vi "Simulation-06.vi"() -> (0 "error out":errorcluster, 3 "success":bool)   [LabVIEW 2020]
uses:
  librarian_class/typedefs/book_state--enum.ctl
  shared/request--enum.ctl
  librarian_class/librarian.lvclass
  client_class/client.lvclass
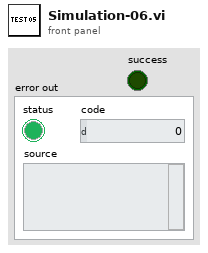
[diagram p1: front panel]
types:
  T1 = typedef "request--enum.ctl" = enum16{"CHECKIN", "CHECKOUT"}
  T2 = typedef "librarian.lvclass/book_state--enum.ctl" = enum16{"CHECKEDIN", "CHECKEDOUT", "DAMAGED"}
  T3 = typedef "message--cluster.ctl" = cluster{"header":string, "cmd":T1, "title":string, "book":string}
  T4 = typedef "librarian.lvclass/lib_map_value--cluster.ctl" = cluster{"book state":T2, "text":string, "hash":string}
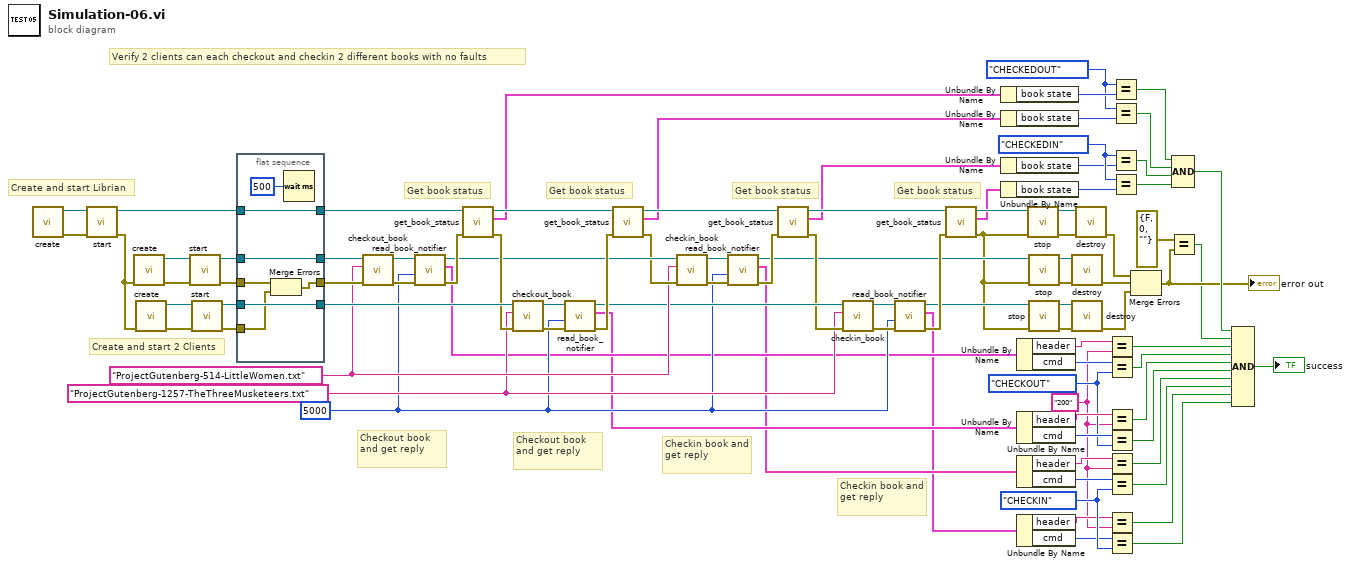
[diagram p0: block diagram]
diagram:
  w23 = request--enum."CHECKIN" ("y")
  w24 = request--enum."CHECKOUT" ("y")
  w18 = "200" ("x")
  w37 = book_state--enum."CHECKEDIN" ("x")
  w38 = book_state--enum."CHECKEDOUT" ("x")
  w58 = 5000 ("timeout in ms (-1)")
  w61 = "ProjectGutenberg-1257-TheThreeMusketeers.txt" ("book title")
  w68 = "ProjectGutenberg-514-LittleWomen.txt" ("book title")
  # "Verify 2 clients can each checkout and checkin 2 different books with no faults"
  # "Get book status"
  # "Get book status"
  # "Get book status"
  # "Get book status"
  # "Checkin book and get reply"
  # "Checkin book and get reply"
  # "Checkout book and get reply"
  # "Checkout book and get reply"
  # "Create and start 2 Clients"
  # "Create and start Librian"
  n1 = call "create.vi"() -> ("error out"=w93:errorcluster, "librarian_sm out"=w94:refnum<class "librarian.lvclass">)  [unwired: 10 in]
  n2 = call "start.vi"("error in (no error)"=w93, "librarian_sm in"=w94) -> ("error out"=w89:errorcluster, "librarian_sm out"=w88:refnum<class "librarian.lvclass">)  [unwired: 8 in]
  n3 = call "create.vi"("error in (no error)"=w89) -> ("error out"=w91:errorcluster, "librarian_sm out"=w92:refnum<class "client.lvclass">)  [unwired: 9 in]
  n4 = call "create.vi"("error in (no error)"=w89) -> ("error out"=w85:errorcluster, "librarian_sm out"=w90:refnum<class "client.lvclass">)  [unwired: 9 in]
  n5 = call "start.vi"("error in (no error)"=w91, "librarian_sm in"=w92) -> ("error out"=w87:errorcluster, "librarian_sm out"=w84:refnum<class "client.lvclass">)  [unwired: 8 in]
  n6 = call "start.vi"("error in (no error)"=w85, "librarian_sm in"=w90) -> ("error out"=w86:errorcluster, "librarian_sm out"=w83:refnum<class "client.lvclass">)  [unwired: 8 in]
  n7 = flat-sequence {
    tunnel: w88 -> [w101]
    tunnel: w87 -> [w97]
    tunnel: w86 -> [w96]
    tunnel: w84 -> [w100]
    tunnel: w83 -> [w99]
    tunnel: [w101] -> w75
    tunnel: [w100] -> w81
    tunnel: [w95] -> w80
    tunnel: [w99] -> w76
    frame #0 {
      n8 = Merge Errors(w97, w96) -> (w95:errorcluster)
      n9 = Wait (ms)(milliseconds to wait=u32 500) -> ()  [unwired: 1 out]
    }
  }
  n10 = call "checkout_book.vi"("error in (no error)"=w80, "book title"=w68, "client in"=w81) -> ("error out"=w79:errorcluster, "client out"=w82:refnum<class "client.lvclass">)  [unwired: 7 in]
  n11 = call "read_book_notifier.vi"("error in (no error)"=w79, "timeout in ms (-1)"=w58, "client in"=w82) -> ("error out"=w74:errorcluster, "msg"=w17:T3, "client out"=w70:refnum<class "client.lvclass">)  [unwired: 6 in]
  n12 = call "get_book_status.vi"("error in (no error)"=w74, "librarian in"=w75) -> ("error out"=w73:errorcluster, "book status"=w40:T4, "librarian out"=w72:refnum<class "librarian.lvclass">)  [unwired: 7 in]
  n13 = call "checkout_book.vi"("error in (no error)"=w73, "book title"=w61, "client in"=w76) -> ("error out"=w78:errorcluster, "client out"=w77:refnum<class "client.lvclass">)  [unwired: 7 in]
  n14 = call "read_book_notifier.vi"("error in (no error)"=w78, "timeout in ms (-1)"=w58, "client in"=w77) -> ("error out"=w71:errorcluster, "msg"=w16:T3, "client out"=w63:refnum<class "client.lvclass">)  [unwired: 6 in]
  n15 = call "get_book_status.vi"("error in (no error)"=w71, "librarian in"=w72) -> ("error out"=w69:errorcluster, "book status"=w39:T4, "librarian out"=w64:refnum<class "librarian.lvclass">)  [unwired: 7 in]
  n16 = call "checkin_book.vi"("error in (no error)"=w69, "book title"=w68, "client in"=w70) -> ("error out"=w67:errorcluster, "client out"=w66:refnum<class "client.lvclass">)  [unwired: 7 in]
  n17 = call "read_book_notifier.vi"("error in (no error)"=w67, "timeout in ms (-1)"=w58, "client in"=w66) -> ("error out"=w65:errorcluster, "msg"=w15:T3, "client out"=w52:refnum<class "client.lvclass">)  [unwired: 6 in]
  n18 = call "get_book_status.vi"("error in (no error)"=w65, "librarian in"=w64) -> ("error out"=w62:errorcluster, "book status"=w34:T4, "librarian out"=w57:refnum<class "librarian.lvclass">)  [unwired: 7 in]
  n19 = call "checkin_book.vi"("error in (no error)"=w62, "book title"=w61, "client in"=w63) -> ("error out"=w60:errorcluster, "client out"=w59:refnum<class "client.lvclass">)  [unwired: 7 in]
  n20 = call "read_book_notifier.vi"("error in (no error)"=w60, "timeout in ms (-1)"=w58, "client in"=w59) -> ("error out"=w56:errorcluster, "msg"=w14:T3, "client out"=w54:refnum<class "client.lvclass">)  [unwired: 6 in]
  n21 = call "get_book_status.vi"("error in (no error)"=w56, "librarian in"=w57) -> ("error out"=w45:errorcluster, "book status"=w33:T4, "librarian out"=w46:refnum<class "librarian.lvclass">)  [unwired: 7 in]
  n22 = Unbundle By Name(w40) -> ("book state"=w42:T2)
  n23 = Unbundle By Name(w39) -> ("book state"=w41:T2)
  n24 = Unbundle By Name(w34) -> ("book state"=w35:T2)
  n25 = Unbundle By Name(w33) -> ("book state"=w36:T2)
  n26 = Unbundle By Name(w17) -> ("header"=w27:string, "cmd"=w28:T1)
  n27 = Unbundle By Name(w16) -> ("header"=w25:string, "cmd"=w26:T1)
  n28 = Unbundle By Name(w15) -> ("header"=w20:string, "cmd"=w19:T1)
  n29 = Unbundle By Name(w14) -> ("header"=w22:string, "cmd"=w21:T1)
  n30 = call "stop.vi"("error in (no error)"=w45, "librarian_sm in"=w46) -> ("error out"=w43:errorcluster, "librarian_sm out"=w47:refnum<class "librarian.lvclass">)  [unwired: 8 in]
  n31 = call "stop.vi"("error in (no error)"=w45, "librarian_sm in"=w52) -> ("error out"=w51:errorcluster, "librarian_sm out"=w53:refnum<class "client.lvclass">)  [unwired: 8 in]
  n32 = call "stop.vi"("error in (no error)"=w45, "librarian_sm in"=w54) -> ("error out"=w50:errorcluster, "librarian_sm out"=w55:refnum<class "client.lvclass">)  [unwired: 8 in]
  n33 = call "destroy.vi"("error in (no error)"=w51, "librarian_sm in"=w53) -> ("error out"=w49:errorcluster)  [unwired: 8 in, 1 out]
  n34 = call "destroy.vi"("error in (no error)"=w50, "librarian_sm in"=w55) -> ("error out"=w48:errorcluster)  [unwired: 8 in, 1 out]
  n35 = call "destroy.vi"("error in (no error)"=w43, "librarian_sm in"=w47) -> ("error out"=w44:errorcluster)  [unwired: 8 in, 1 out]
  n36 = Equal?(x=w27, y=w18) -> (x = y?=w13:bool)
  n37 = Equal?(x=w28, y=w24) -> (x = y?=w12:bool)
  n38 = Equal?(x=w25, y=w18) -> (x = y?=w11:bool)
  n39 = Equal?(x=w26, y=w24) -> (x = y?=w10:bool)
  n40 = Equal?(x=w20, y=w18) -> (x = y?=w9:bool)
  n41 = Equal?(x=w19, y=w23) -> (x = y?=w8:bool)
  n42 = Equal?(x=w22, y=w18) -> (x = y?=w7:bool)
  n43 = Equal?(x=w21, y=w23) -> (x = y?=w6:bool)
  n44 = Equal?(x=w38, y=w42) -> (x = y?=w29:bool)
  n45 = Equal?(x=w38, y=w41) -> (x = y?=w30:bool)
  n46 = Equal?(x=w37, y=w35) -> (x = y?=w31:bool)
  n47 = Equal?(x=w37, y=w36) -> (x = y?=w32:bool)
  n48 = Merge Errors(w44, w49, w48) -> (w3:errorcluster)
  "error out" <- w3
  n49 = Equal?(x=errorcluster {"status"=FALSE, "code"=0, "source"=""} ("y"), y=w3) -> (x = y?=w2:bool)
  n50 = Compound Arithmetic op=AND(w29, w30, w31, w32) -> (w5:bool)
  n51 = Compound Arithmetic op=AND(w5, w2, w13, w12, w11, w10, w9, w8, w7, w6) -> (→"success":bool)
